vi "Digital has been set.vi"(8 "error in":errorcluster, 10 "Digital Signal":T1={"DAQ Board Name"="DAQ_Simu1", "Port Digitales"=[], "rate"=1000.0, "Tiempo"=100}) -> (0 "error out":errorcluster)   [LabVIEW 2020, in "Settings.lvlib"]
doc: "digital signal has been set\n_____\nCreated using Delacor QMH Event Scripter 6.0.0.121."
uses:
  Settings.lvlib
  Digital typeSignal--cluster.ctl
  Digital has been set Argument--cluster.ctl
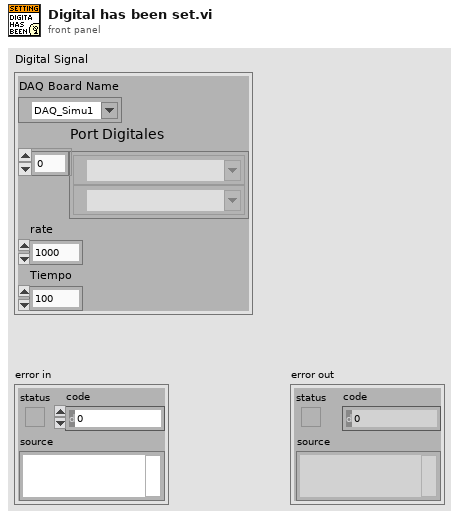
[diagram p1: front panel]
types:
  T1 = typedef "Digital typeSignal--cluster.ctl" = cluster{"DAQ Board Name":tag, "Port Digitales":tag[], "rate":dbl, "Tiempo":i32}
  T2 = typedef "Settings.lvlib/Digital has been set Argument--cluster.ctl" = cluster{"Digital Signal":T1}
  T3 = typedef "Settings.lvlib/Broadcast Events--cluster.ctl" = cluster{"Module Did Init":refnum<user-event>, "Status Updated":refnum<user-event>, "Error Reported":refnum<user-event>, "Module Did Stop":refnum<user-event>, "Update Module Execution Status":refnum<user-event>, "Config has been set":refnum<user-event>, "Prueba has been set":refnum<user-event>, "Digital has been set":refnum<user-event>}
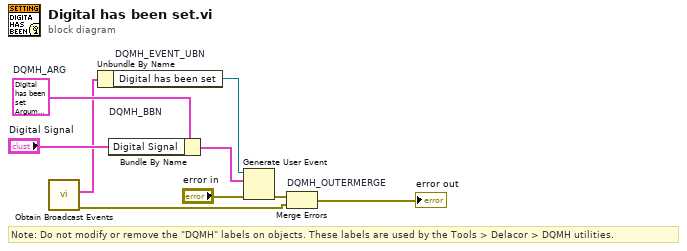
[diagram p0: block diagram]
diagram:
  w4 = T2 {"Digital Signal"={"DAQ Board Name"="DAQ_Simu1", "Port Digitales"=[], "rate"=1000.0, "Tiempo"=100}}  # DQMH_ARG
  # "Note: Do not modify or remove the \"DQMH\" labels on objects. These labels are used by the Tools > Delacor > DQMH utilities."
  n1 = call "Obtain Broadcast Events.vi"() -> ("error out"=w2:errorcluster, "Settings Broadcast Events"=w1:T3)  [unwired: 10 in]
  n2 = Unbundle By Name "DQMH_EVENT_UBN"(w1) -> ("Digital has been set"=w6:refnum<user-event>)
  n3 = Bundle By Name "DQMH_BBN"(cluster=w4, "Digital Signal"="Digital Signal") -> (w7:T2)
  n4 = Generate User Event(user event=w6, event data cluster=w7, error in="error in") -> (error out=w5:errorcluster)  [unwired: 1 in, 1 out]
  n5 = Merge Errors "DQMH_OUTERMERGE"(w5, w2) -> (→"error out":errorcluster)
